vi "3D_Traverse_move.vi"(0 "Mode":T3=enum."Read traverse position", 1 "Route Checking?":bool=TRUE, 2 "Row Number":i32=-1, 5 "Position":dbl[](array[numeric])=[0.0, 0.0, 0.0] format="%#.2f", 7 "Work in Tunnel Coordinates":T1, 11 "Simulate/Run":T2=enum."Run VI", 12 "Traverse name":string, 13 "Backlash Compensation?":bool=TRUE, 14 "Currently on Point":i32=-1) -> (3 "Model Rotation (deg)":dbl format="%#.2f", 4 "Trav Position achieved":dbl[](array[numeric]) format="%#.2f", 15 "Error String":string)   [LabVIEW 2010]
uses:
  Trav_mode.ctl
  Controls/User_Specific_mode.ctl
  Controls/Tunnel_Coordinates.ctl
  Route mapping/Route_Display_Mode.ctl
  Controls/In_Range.ctl
  Globals/Trav_pos_global.vi
  Globals/Constants_global.vi
  Route mapping/Route_mapping_global.vi
panel:
  in  "Position Increment":dbl[](array[numeric])=[0.0, 0.0, 0.0] step=0.1 format="%#.2f"
  out "Traverses Available":string[](array[string])
  in  "Traverse":u16(ring) items=["A_Tunnel", "Aero_Laser", "Aero_ThroughWall", "Aero_Tunnel", "Angle_Calibrator", "B_Tunnel", "D_Tunnel", "Dummy_Traverse", "EnFlo_Stack", "EnFlo_Tunnel", "EnFlo_Turntable", "Laser_Meas_Traverse", "mohd_setup", "Paul_Desk_Test", "PIV_Traverse"]
  # "X                Y                   Z"
  # "X                Y                   Z"
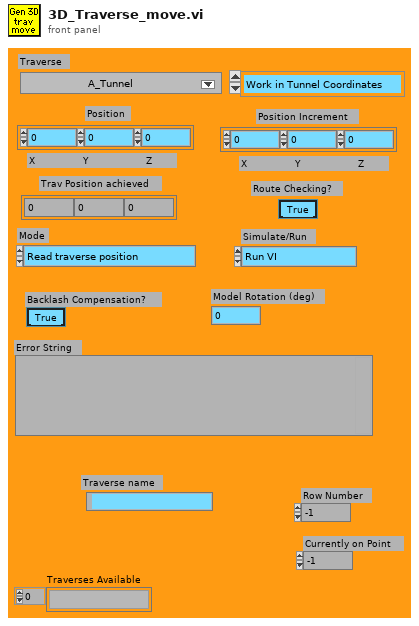
[diagram p1: front panel]
types:
  T1 = typedef "Tunnel_Coordinates.ctl" = enum16{"Work in Tunnel Coordinates", "Work in Model Coordinates"}
  T2 = typedef "User_Specific_mode.ctl" = enum16{"Check VI only", "Run VI"}
  T3 = typedef "Trav_mode.ctl" = enum16{"Move traverse", "Read traverse position", "Teach Position"}
  T4 = enum16{"To Traverse Coordinates", "To User Coordinates"}
  T5 = typedef "Route_Display_Mode.ctl" = enum16{"Display View Always", "Display View on Crash"}
  T6 = typedef "In_Range.ctl" = enum16{"%", "±", "% & ±"}
  T7 = typedef "Box_size.ctl" = cluster{"Max":dbl, "Min":dbl}[]
  T8 = typedef "Exclude_cluster.ctl" = cluster{"Sizes":T7, "Name":string, "Exclude Type":T9}
  T9 = typedef "Exclusion_type.ctl" = enum16{"Exclude completely", "Allow only vertical moves"}
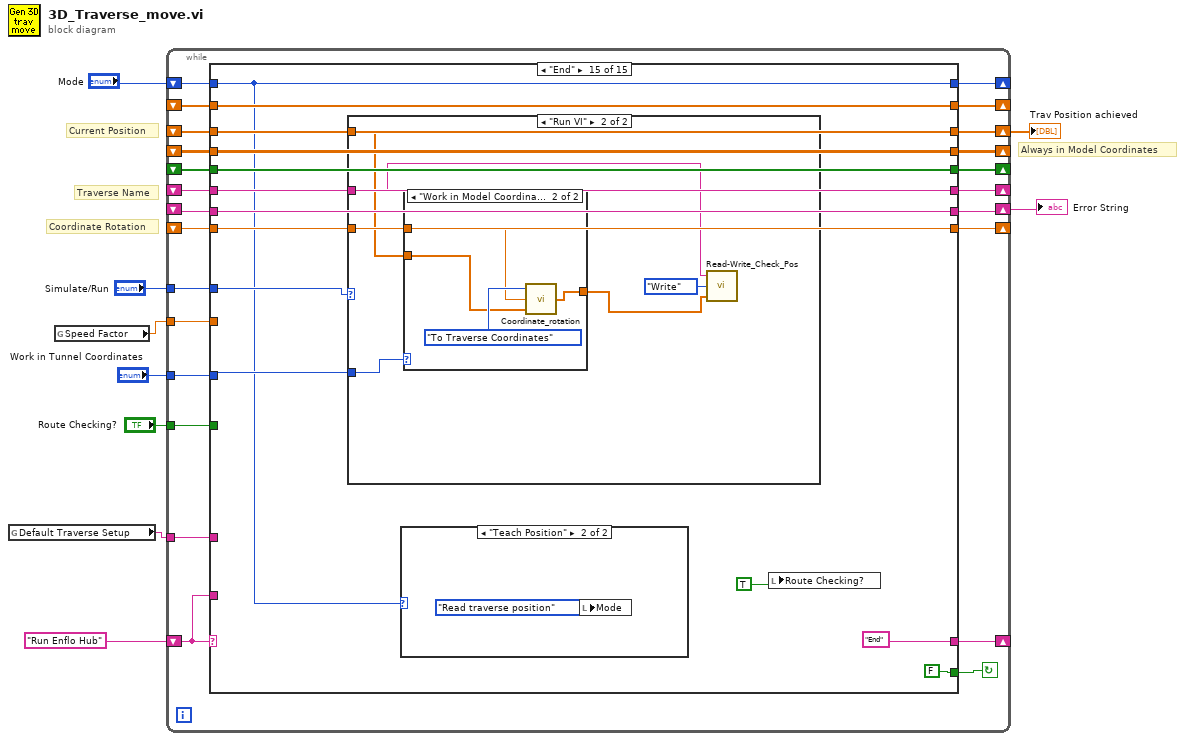
[diagram p0: block diagram]
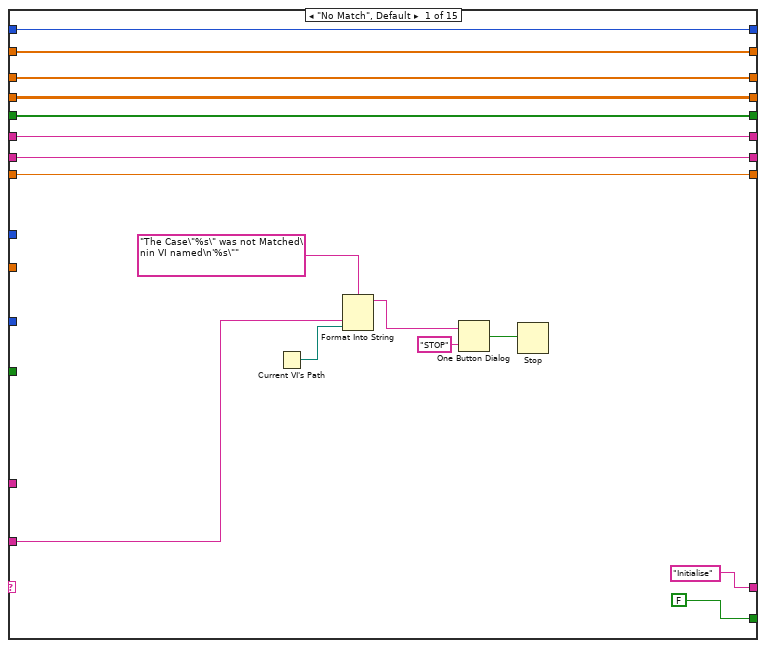
[diagram p2: hidden frame]
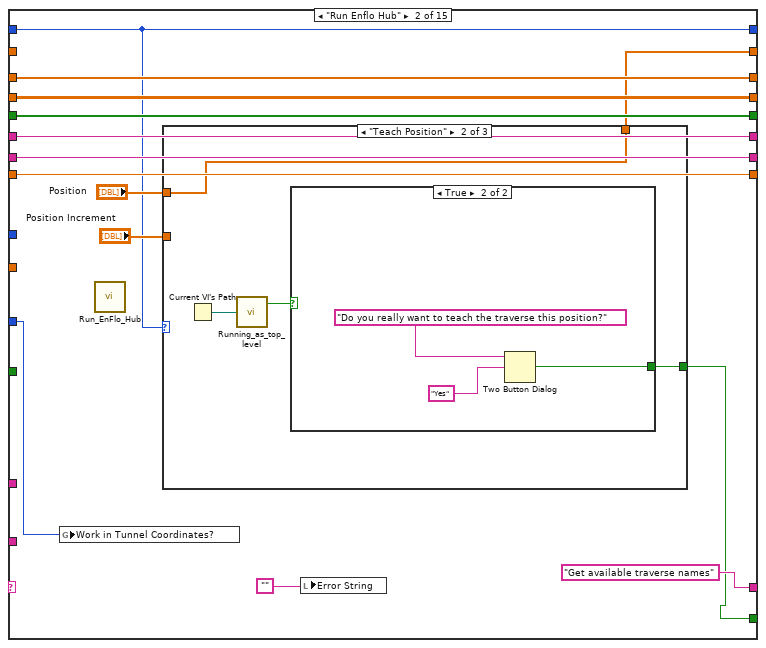
[diagram p3: hidden frame]
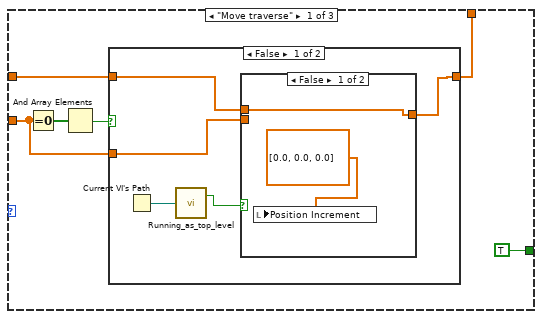
[diagram p4: hidden frame]
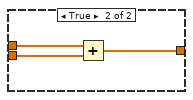
[diagram p5: hidden frame]
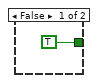
[diagram p7: hidden frame]
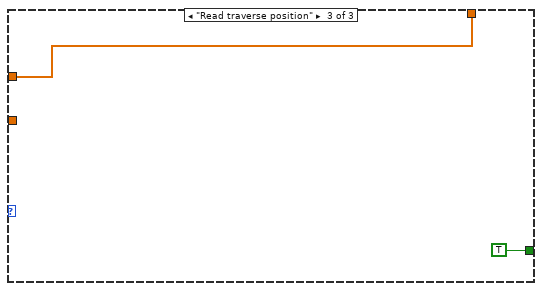
[diagram p8: hidden frame]
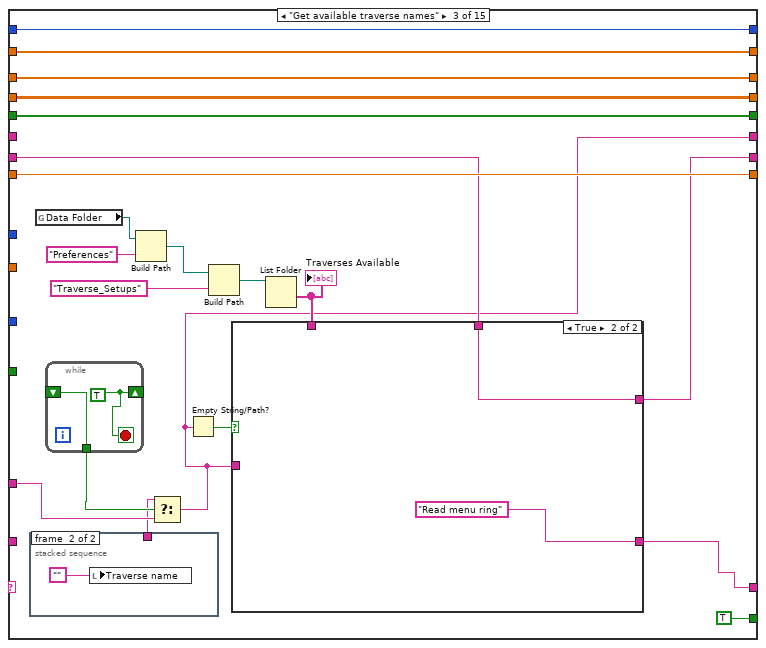
[diagram p9: hidden frame]
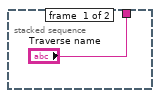
[diagram p10: hidden frame]
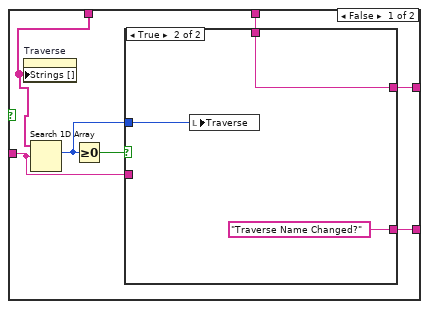
[diagram p11: hidden frame]
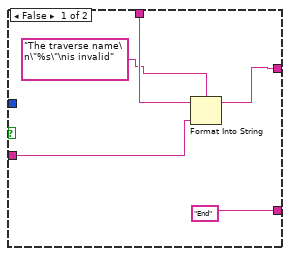
[diagram p12: hidden frame]
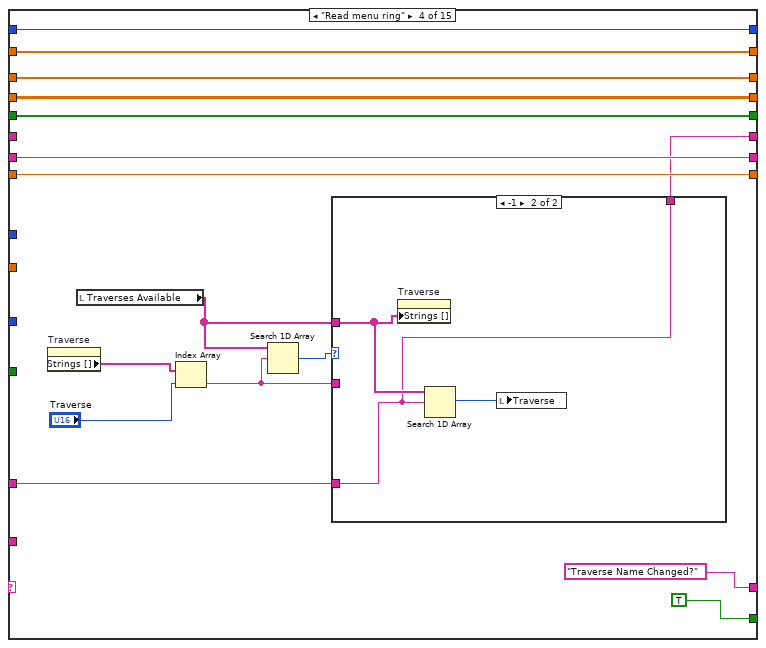
[diagram p13: hidden frame]
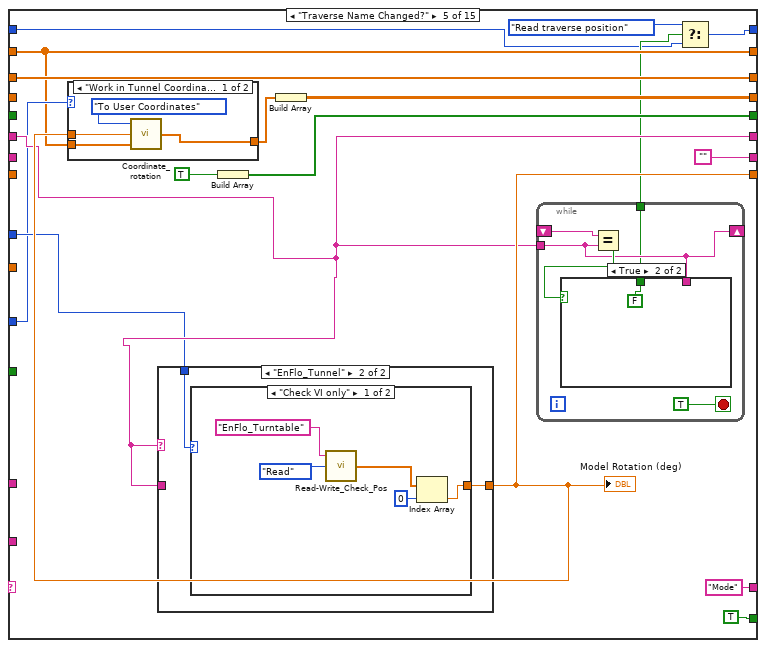
[diagram p15: hidden frame]
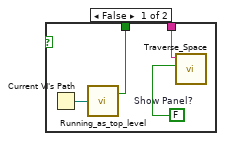
[diagram p17: hidden frame]
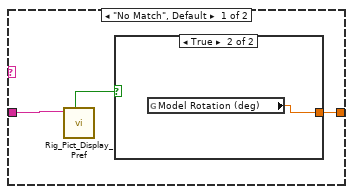
[diagram p18: hidden frame]
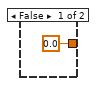
[diagram p19: hidden frame]
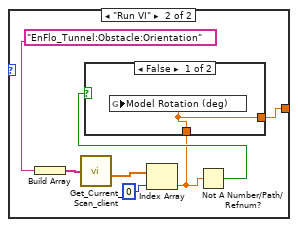
[diagram p20: hidden frame]
diagram:
  # "Always in Model Coordinates"
  # "Current Position"
  # "Coordinate Rotation"
  # "Traverse Name"
  n1 = global read "Trav_pos_global.vi" "Default Traverse Setup"() -> (w2:string)
  n2 = global read "Trav_pos_global.vi" "Speed Factor"() -> (w6:dbl)
  n3 = while {
    shift-left: "Run Enflo Hub" -> [w31]
    shift-right: [w32] -> _
    shift-right: [w29] -> _
    shift-left: _ -> [w27]
    tunnel: "Simulate/Run" -> [w30]
    shift-right: [w28] -> w7
    shift-left: _ -> [w26]
    shift-right: [w24] -> _
    shift-left: _ -> [w25]
    shift-right: [w19] -> _
    shift-left: _ -> [w18]
    shift-right: [w21] -> _
    shift-left: _ -> [w20]
    shift-right: [w22] -> w3
    shift-left: _ -> [w23]
    tunnel: w6 -> [w17]
    tunnel: "Work in Tunnel Coordinates" -> [w16]
    tunnel: "Route Checking?" -> [w15]
    tunnel: w2 -> [w14]
    shift-right: [w13] -> _
    shift-left: _ -> [w12]
    shift-right: [w10] -> _
    shift-left: "Mode" -> [w11]
    stop <- w33 continue-if-true
    n4 = case shown="\"End\"" w31 {
      tunnel: [FALSE w55 TRUE TRUE TRUE TRUE w266 TRUE ("T button?") TRUE w352 w372 TRUE TRUE TRUE FALSE] -> w33
      tunnel: ["Initialise" "Get available traverse names" w101 "Traverse Name Changed?" "Mode" w215 w255 "Perform Route Check" w316 "Display Traverse Views" w379 "Update Position Globals" "Tidy up" "End" "End"] -> w32
      tunnel: w31 -> [w44 _ _ _ _ _ _ _ _ _ _ _ _ _ _]
      tunnel: w30 -> [_ _ _ _ w159 w216 w260 _ w312 _ w377 _ _ _ w510]
      tunnel: [w41 w62 w94 w133 w160 w207 w268 w292 w311 w359 w384 w420 w445 w462 w506] -> w29
      tunnel: [w40 w61 w99 w146 "" w217 w267 "" w321 w349 w381 w409 w448 w464 w513] -> w28
      tunnel: w27 -> [w41 w62 _ _ w160 w207 w268 w292 w311 w359 w384 w420 w445 w462 w506]
      tunnel: w26 -> [w40 w61 w98 w146 _ w217 _ _ _ w350 w381 _ w448 w465 w513]
      tunnel: w25 -> [w39 w60 w111 w145 _ w218 w264 w295 w307 w358 w388 w416 w447 w468 w507]
      tunnel: [w39 w60 w111 w145 w162 w218 w264 w295 w307 w358 w388 w416 w447 w468 w507] -> w24
      tunnel: w23 -> [w38 w59 w110 w144 w165 w209 w261 _ w319 w357 w387 _ w444 w466 w508]
      tunnel: [w38 w59 w110 w144 w165 w209 w262 w294 w320 w357 w387 w414 w444 w466 w508] -> w22
      tunnel: [w37 w58 w109 w143 w166 w220 w270 w299 w318 w356 w385 w418 w449 w469 w514] -> w21
      tunnel: w20 -> [w37 w58 w109 w143 _ w220 w270 w299 _ w356 w385 w418 w449 w469 w514]
      tunnel: [w36 w57 w108 w142 w163 w219 w269 w298 w323 w355 w386 w412 w450 w470 w515] -> w19
      tunnel: w18 -> [w36 w57 w108 w142 _ w219 w269 w298 _ w355 w386 w412 w450 w470 w515]
      tunnel: w17 -> [_ _ _ _ _ _ _ _ _ _ _ w419 _ _ _]
      tunnel: w16 -> [_ w54 _ _ w158 w211 w265 w296 w329 _ _ w417 _ _ w509]
      tunnel: w15 -> [_ _ _ _ _ w212 _ _ _ _ _ w408 _ _ _]
      tunnel: w14 -> [_ _ w95 w137 _ _ _ _ _ _ _ _ _ _ _]
      tunnel: [w35 w53 w92 w135 w157 w208 w254 w293 w306 w348 w371 w407 w446 w461 w511] -> w13
      tunnel: w12 -> [w35 _ w92 w135 w157 w208 w254 w293 w306 w348 w371 w407 w446 w461 w511]
      tunnel: w11 -> [w34 w50 w91 w134 w153 w206 w253 w288 w305 w347 w370 w406 w443 w460 w505]
      tunnel: [w34 w50 w91 w134 w154 w206 w253 w288 w305 w347 w370 w406 w443 w460 w505] -> w10
      frame "No Match", Default {
        n5 = Current VI's Path() -> (path=w43:path)
        n6 = Format Into String(format string="The Case\"%s\" was not Matched\nin VI named\n'%s\"" ("Format String"), w44, w43) -> (resulting string=w47:string)  [unwired: 2 in, 1 out]
        n7 = One Button Dialog(message=w47, button name ("OK")="STOP") -> (true=w45:bool)
        n8 = Stop(stop? (T)=w45) -> ()
      }
      frame "Run Enflo Hub" {
        n9 = global write "Trav_pos_global.vi" "Work in Tunnel Coordinates?"(w54) -> ()
        n10 = call "Run_EnFlo_Hub.vi"() -> ()  [unwired: 8 out]
        n11 = case shown="\"Teach Position\"" w50 {
          tunnel: [TRUE ("T button?") w82 TRUE ("T button?")] -> w55
          tunnel: [w66 w81 w90] -> w53
          tunnel: "Position" -> [w65 w81 w90]
          tunnel: "Position Increment" -> [w64 _ _]
          frame "Move traverse" {
            n12 = Equal To 0?(x=w64) -> (x = 0?=w68:bool[])
            n13 = And Array Elements(Boolean array=w68) -> (logical AND=w67:bool)
            n14 = case shown="False" w67 {
              tunnel: [w70 w80] -> w66
              tunnel: w65 -> [w72 w80]
              tunnel: w64 -> [w71 _]
              frame False {
                n15 = Current VI's Path() -> (path=w74:path)
                n16 = call "Running_as_top_level.vi"("Vi path name"=w74) -> ("Top Level"=w73:bool)  [unwired: 1 out]
                n17 = case shown="False" w73 {
                  tunnel: w72 -> [w76 w79]
                  tunnel: w71 -> [_ w78]
                  tunnel: [w76 w77] -> w70
                  frame False {
                    n18 = local write "Position Increment"(dbl[] [0.0, 0.0, 0.0] ("Position Increment")) -> ()
                  }
                  frame True {
                    n19 = Add(x=w79, y=w78) -> (x+y=w77:dbl[])
                  }
                }
              }
              frame True {
              }
            }
          }
          frame "Teach Position" {
            n20 = Current VI's Path() -> (path=w84:path)
            n21 = call "Running_as_top_level.vi"("Vi path name"=w84) -> ("Top Level"=w83:bool)  [unwired: 1 out]
            n22 = case shown="True" w83 {
              tunnel: [TRUE ("T button?") w86] -> w82
              frame False {
              }
              frame True {
                n23 = Two Button Dialog(message="Do you really want to teach the traverse this position?", 2:"Yes" ("T button name (\"OK\")")) -> (T button?=w86:bool)  [unwired: 1 out]
              }
            }
          }
          frame "Read traverse position" {
          }
        }
        n24 = local write "Error String"("") -> ()
      }
      frame "Get available traverse names" {
        n25 = stacked-sequence {
          tunnel: ["Traverse name" _] -> w93
          frame #0 {
          }
          frame #1 {
            n26 = local write "Traverse name"("") -> ()
          }
        }
        n27 = global read "Constants_global.vi" "Data Folder"() -> (w104:path)
        n28 = while {
          shift-right: [w114] -> _
          shift-left: _ -> [w115]
          tunnel: [w115] -> w96
          stop <- w114 stop-if-true
          w114 = TRUE
        }
        n29 = Build Path(base path=w104, name or relative path="Preferences") -> (appended path=w106:path)
        n30 = Select(t=w93, s=w96, f=w95) -> (s? t:f=w94:string)
        n31 = Empty String/Path?(string/path=w94) -> (empty?=w102:bool)
        n32 = Build Path(base path=w106, name or relative path="Traverse_Setups") -> (appended path=w107:path)
        n33 = List Folder(path=w107) -> (folder names=w100:string[])  [unwired: 1 in, 5 out]
        "Traverses Available" <- w100
        n34 = case shown="True" w102 {
          tunnel: [w119 "Read menu ring"] -> w101
          tunnel: w100 -> [w116 _]
          tunnel: w94 -> [w122 _]
          tunnel: [w121 w131] -> w99
          tunnel: w98 -> [w120 w131]
          frame False {
            n35 = property on="Traverse" class="Ring (strict)"("Strings []"=w116) -> ()  [unwired: 2 in, 2 out]
            n36 = Search 1D Array(1D array=w116, element=w122) -> (index of element=w117:i32)  [unwired: 1 out]
            n37 = Greater Or Equal To 0?(x=w117) -> (x >= 0?=w118:bool)
            n38 = case shown="True" w118 {
              tunnel: w122 -> [w127 _]
              tunnel: [w124 w130] -> w121
              tunnel: w120 -> [w126 w130]
              tunnel: ["End" "Traverse Name Changed?"] -> w119
              tunnel: w117 -> [_ w128]
              frame False {
                n39 = Format Into String(format string="The traverse name\n\"%s\"\nis invalid", initial string=w126, w127) -> (resulting string=w124:string)  [unwired: 1 in, 1 out]
              }
              frame True {
                n40 = local write "Traverse"(w128) -> ()
              }
            }
          }
          frame True {
          }
        }
      }
      frame "Read menu ring" {
        n41 = property on="Traverse" class="Ring (strict)"() -> ("Strings []"=w141:string[])  [unwired: 2 in, 2 out]
        n42 = local read "Traverses Available"() -> (w138:string[])
        n43 = Index Array(array=w141, index="Traverse") -> (element=w136:string)
        n44 = Search 1D Array(1D array=w138, element=w136) -> (index of element=w139:i32)  [unwired: 1 out]
        n45 = case shown="-1" w139 {
          tunnel: w138 -> [_ w152]
          tunnel: w137 -> [_ w150]
          tunnel: [w149 w150] -> w133
          tunnel: w136 -> [w149 _]
          frame 0, Default {
          }
          frame -1 {
            n46 = property on="Traverse" class="Ring (strict)"("Strings []"=w152) -> ()  [unwired: 2 in, 2 out]
            n47 = Search 1D Array(1D array=w152, element=w150) -> (index of element=w151:i32)  [unwired: 1 out]
            n48 = local write "Traverse"(w151) -> ()
          }
        }
      }
      frame "Traverse Name Changed?" {
        n49 = case shown="\"EnFlo_Tunnel\"" w160 {
          tunnel: [w185 w191] -> w162
          tunnel: w159 -> [_ w190]
          tunnel: w160 -> [w187 _]
          frame "No Match", Default {
            n50 = call "Rig_Pict_Display_Pref.vi"("Traverse Name"=w187) -> ("Co-ordinate Transform"=w186:bool)  [unwired: 7 out]
            n51 = case shown="True" w186 {
              tunnel: [0.0 ("Model Rotation (deg)") w189] -> w185
              frame False {
              }
              frame True {
                n52 = global read "Trav_pos_global.vi" "Model Rotation (deg)"() -> (w189:dbl)
              }
            }
          }
          frame "EnFlo_Tunnel" {
            n53 = case shown="\"Check VI only\"" w190 {
              tunnel: [w192 w197] -> w191
              frame "Check VI only" {
                n54 = call "Read-Write_Check_Pos.vi"("Mode"=enum16{"Read", "Write"}."Read", "Traverse Name"="EnFlo_Turntable") -> ("Position Output"=w194:dbl[])  [unwired: 1 in]
                n55 = Index Array(array=w194, index=0) -> (element=w192:dbl)
              }
              frame "Run VI" {
                n56 = Build Array("EnFlo_Tunnel:Obstacle:Orientation") -> (w202:string[])
                n57 = call "Get_Current_Scan_client.vi"("ADAM Ch Names"=w202) -> ("Numerical Values"=w201:dbl[])  [unwired: 3 out]
                n58 = Index Array(array=w201, index=0) -> (element=w198:dbl)
                n59 = Not A Number/Path/Refnum?(number/path/refnum=w198) -> (NaN/Path/Refnum?=w199:bool)
                n60 = case shown="False" w199 {
                  tunnel: w198 -> [w204 _]
                  tunnel: [w204 w205] -> w197
                  frame False {
                    n61 = global write "Trav_pos_global.vi" "Model Rotation (deg)"(w204) -> ()
                  }
                  frame True {
                    n62 = global read "Trav_pos_global.vi" "Model Rotation (deg)"() -> (w205:dbl)
                  }
                }
              }
            }
          }
        }
        "Model Rotation (deg)" <- w162
        n63 = case shown="\"Work in Tunnel Coordinates\"" w158 {
          tunnel: w157 -> [w172 w174]
          tunnel: [w171 w174] -> w161
          tunnel: w162 -> [w170 _]
          frame "Work in Tunnel Coordinates" {
            n64 = call "Coordinate_rotation.vi"("Input Position"=w172, "Coordinate rotation (deg)"=w170, "Mode"=T4."To User Coordinates") -> ("Output Position"=w171:dbl[])
          }
          frame "Work in Model Coordinates" {
          }
        }
        n65 = Build Array(TRUE) -> (w163:bool[])
        n66 = Build Array(w161) -> (w166:dbl[][])
        n67 = while {
          shift-right: [w176] -> _
          shift-left: _ -> [w178]
          tunnel: w160 -> [w176]
          tunnel: [w175] -> w156
          stop <- TRUE stop-if-true
          n68 = Equal?(x=w178, y=w176) -> (x = y?=w177:bool)
          n69 = case shown="True" w177 {
            tunnel: w176 -> [w182 _]
            tunnel: [w180 FALSE ("Top Level")] -> w175
            frame False {
              w183 = FALSE  # Show Panel?
              n70 = Current VI's Path() -> (path=w181:path)
              n71 = call "Running_as_top_level.vi"("Vi path name"=w181) -> ("Top Level"=w180:bool)  [unwired: 1 out]
              n72 = call "Traverse_Space.vi"("Show Panel?"=w183, "Traverse Setup"=w182) -> ()  [unwired: 1 in, 8 out]
            }
            frame True {
            }
          }
        }
        n73 = Select(t=Trav_mode."Read traverse position" ("Mode"), s=w156, f=w153) -> (s? t:f=w154:T3)
      }
      frame "Mode" {
        n74 = while {
          shift-right: [w224] -> _
          shift-left: _ -> [w223]
          tunnel: w211 -> [w224]
          tunnel: [w222] -> w210
          stop <- TRUE stop-if-true
          n75 = Equal?(x=w223, y=w224) -> (x = y?=w222:bool)
        }
        n76 = case shown="\"Run VI\"" w216 {
          tunnel: w206 -> [_ w232]
          tunnel: [w226 w231] -> w215
          tunnel: "Execute case" -> [_ w230]
          tunnel: "Read Current Position" -> [w226 w229]
          tunnel: w212 -> [_ w228]
          tunnel: w210 -> [_ _]
          tunnel: w207 -> [_ w227]
          frame "Check VI only" {
          }
          frame "Run VI" {
            n77 = case shown="\"Move traverse\"" w232 {
              tunnel: [w235 w252] -> w231
              tunnel: w230 -> [w234 w252]
              tunnel: w229 -> [w233 _]
              tunnel: w228 -> [w236 _]
              tunnel: w227 -> [w237 _]
              frame "Move traverse" {
                n78 = case shown="True" w236 {
                  tunnel: w237 -> [_ w248]
                  tunnel: [w238 w242] -> w235
                  tunnel: w234 -> [w238 _]
                  tunnel: w233 -> [_ w240]
                  frame False {
                  }
                  frame True {
                    n79 = global read "Constants_global.vi" "Traverse folder"() -> (w249:path)
                    n80 = Build Path(base path=w249, name or relative path=w248) -> (appended path=w251:path)
                    n81 = Build Path(base path=w251, name or relative path="Traverse_Pos.xls" ("Substring")) -> (appended path=w247:path)
                    n82 = File/Directory Info(path=w247) -> (last mod=w245:timestamp)  [unwired: 1 in, 6 out]
                    n83 = Get Date/Time In Seconds() -> (seconds since 1Jan1904=w246:timestamp)
                    n84 = Subtract(x=w246, y=w245) -> (x-y=w244:dbl)
                    n85 = Greater?(x=w244, y=40.0) -> (0:w241:bool)
                    n86 = Select(t=w240, s=w241, f="Quick Read from file") -> (s? t:f=w242:string)
                  }
                }
              }
              frame "Read traverse position", Default {
              }
            }
          }
        }
      }
      frame "Read Current Position" {
        n87 = case shown="\"Run VI\"" w260 {
          tunnel: w268 -> [w271 w280]
          tunnel: ["" w282] -> w267
          tunnel: w264 -> [_ w275]
          tunnel: [w272 w281] -> w263
          tunnel: w261 -> [_ w277]
          frame "Check VI only" {
            n88 = call "Read-Write_Check_Pos.vi"("Mode"=enum16{"Read", "Write"}."Read", "Traverse Name"=w271) -> ("Position Output"=w272:dbl[])  [unwired: 1 in]
          }
          frame "Run VI" {
            w279 = FALSE  # Route Checking?
            w278 = FALSE  # Backlash Compensation?
            n89 = call "TraverseControl.vi"("Mode"=Trav_mode."Read traverse position", "Route Checking?"=w279, "Traverse Name"=w280, "Coordinate rotation (deg)"=w275, "Position input XYZ"=w277, "Backlash Compensation?"=w278) -> ("Position Output XYZ"=w281:dbl[], "Error String"=w282:string)  [unwired: 1 in, 7 out]
          }
        }
        n90 = Equal?(x=Trav_mode."Read traverse position" ("Mode"), y=w253) -> (x = y?=w258:bool)
        n91 = case shown="\"Work in Model Coordinates\"" w265 {
          tunnel: w263 -> [w283 w286]
          tunnel: [w283 w285] -> w262
          tunnel: w264 -> [_ w284]
          frame "Work in Tunnel Coordinates" {
          }
          frame "Work in Model Coordinates" {
            n92 = call "Coordinate_rotation.vi"("Input Position"=w286, "Coordinate rotation (deg)"=w284, "Mode"=T4."To User Coordinates") -> ("Output Position"=w285:dbl[])
          }
        }
        n93 = Empty String/Path?(string/path=w267) -> (empty?=w266:bool)
        n94 = Select(t="Update Position Globals", s=w258, f="Perform Route Check") -> (s? t:f=w255:string)
      }
      frame "Quick Read from file" {
        n95 = call "Read_Traverse_Pos_File.vi"("Traverse Name"=w292) -> ("Tunnel Coordinates"=w291:dbl[])
        n96 = case shown="\"Work in Model Coordinates\"" w296 {
          tunnel: w291 -> [w300 w303]
          tunnel: [w300 w302] -> w294
          tunnel: w295 -> [_ w301]
          frame "Work in Tunnel Coordinates" {
          }
          frame "Work in Model Coordinates" {
            n97 = call "Coordinate_rotation.vi"("Input Position"=w303, "Coordinate rotation (deg)"=w301, "Mode"=T4."To User Coordinates") -> ("Output Position"=w302:dbl[])
          }
        }
      }
      frame "Perform Route Check" {
        n98 = case shown="\"Work in Tunnel Coordinates\"" w329 {
          tunnel: w307 -> [w343 _]
          tunnel: w306 -> [w339 w345]
          tunnel: w319 -> [w342 w346]
          tunnel: [w341 w345] -> w310
          tunnel: [w340 w346] -> w322
          frame "Work in Tunnel Coordinates" {
            w344 = T4."To User Coordinates" ("Mode")
            n99 = call "Coordinate_rotation.vi"("Input Position"=w342, "Coordinate rotation (deg)"=w343, "Mode"=w344) -> ("Output Position"=w340:dbl[])
            n100 = call "Coordinate_rotation.vi"("Input Position"=w339, "Coordinate rotation (deg)"=w343, "Mode"=w344) -> ("Output Position"=w341:dbl[])
          }
          frame "Work in Model Coordinates" {
          }
        }
        n101 = global read "Route_mapping_global.vi" "Entire Space"() -> (w328:T7)
        n102 = global read "Route_mapping_global.vi" "Exclude Array"() -> (w326:T8[])
        n103 = global read "Route_mapping_global.vi" "Probe Volume"() -> (w327:T7)
        n104 = call "Check_with_Jump.vi"("Rotation (deg)"=w307, "Simulate/Run"=w312, "Exclude Array"=w326, "Traverse Name"=w311, "Probe Volume"=w327, "Entire Space"=w328, "New Position"=w310, "Current position"=w322) -> ("Steps"=w318:dbl[][], "Error Comments"=w321:string)  [unwired: 2 out]
        n105 = Array Size(array=w318) -> (size(s)=w325:i32[])
        n106 = Empty String/Path?(string/path=w321) -> (empty?=w313:bool)
        n107 = case shown="True" w313 {
          tunnel: [w337 w338] -> w320
          tunnel: w319 -> [w337 _]
          tunnel: w306 -> [_ w338]
          frame False {
          }
          frame True {
          }
        }
        n108 = Index Array(array=w325, index=0) -> (element=w308:i32)
        n109 = case shown="3, Default" w308 {
          tunnel: [w331 w333 w336] -> w323
          tunnel: "Backlash Compensation?" -> [w330 w332 w334]
          frame 1 {
            n110 = Build Array(w330) -> (w331:bool[])
          }
          frame 2 {
            n111 = Build Array(w332, w332) -> (w333:bool[])
          }
          frame 3, Default {
            n112 = Build Array(FALSE, w334, w334) -> (w336:bool[])
          }
        }
        n113 = Select(t="Display Traverse Views", s=w313, f="Route Error") -> (s? t:f=w316:string)
      }
      frame "Route Error" {
        n114 = global read "Trav_pos_global.vi" "Jump Bad Positions?"() -> (w354:bool)
        n115 = case shown="True" w354 {
          tunnel: w348 -> [_ w362]
          tunnel: [TRUE w361] -> w352
          frame False {
          }
          frame True {
            n116 = Current VI's Path() -> (path=w364:path)
            n117 = call "Running_as_top_level.vi"("Vi path name"=w364) -> ("Top Level"=w363:bool)  [unwired: 1 out]
            n118 = case shown="False" w363 {
              tunnel: w362 -> [w366 _]
              tunnel: [FALSE TRUE] -> w361
              frame False {
                n119 = global read "Trav_pos_global.vi" "Jumped Positions"() -> (w365:dbl[][])
                n120 = Build Array (concatenate)(w366, w365) -> (w368:dbl[][])
                n121 = global write "Trav_pos_global.vi" "Jumped Positions"(w368) -> ()
              }
              frame True {
              }
            }
          }
        }
        n122 = Concatenate Strings("Route Checking Error\n" ("string"), w350) -> (w349:string)
      }
      frame "Display Traverse Views" {
        n123 = global read "Route_mapping_global.vi" "Display Mode"() -> (w383:T5)
        n124 = Equal?(x=w377, y=User_Specific_mode."Check VI only" ("Simulate/Run")) -> (x = y?=w376:bool)
        n125 = Empty String/Path?(string/path=w381) -> (empty?=w372:bool)
        n126 = Equal?(x=w383, y=Route_Display_Mode."Display View Always" ("Display Mode")) -> (x = y?=w380:bool)
        n127 = Not(x=w372) -> (.not. x?=w373:bool)
        n128 = Or(x=w380, y=w373) -> (x .or. y?=w375:bool)
        n129 = And(x=w376, y=w375) -> (x .and. y?=w374:bool)
        n130 = case shown="True" w374 {
          tunnel: w385 -> [_ w397]
          tunnel: w384 -> [_ w396]
          tunnel: w381 -> [_ w393]
          tunnel: w372 -> [_ w391]
          frame False {
          }
          frame True {
            n131 = Not(x=w391) -> (.not. x?=w392:bool)
            n132 = for {
              tunnel: w397 -> [w404] mode=indexing
              tunnel: w396 -> [w403]
              tunnel: "Currently on Point" -> [w402]
              tunnel: "Row Number" -> [w401]
              tunnel: w393 -> [w400]
              tunnel: w392 -> [w398]
              n133 = Build Array(w404) -> (w405:dbl[][])
              n134 = call "Display_Trav_Views.vi"("Current Probe Position"=w405, "Traverse Name"=w403, "Currently on point"=w402, "Open Front Panel"=TRUE, "Error Comments"=w400, "Crash?"=w398, "Row Number"=w401) -> ()  [unwired: 4 out]
            }
          }
        }
        n135 = case shown="\"Check VI only\"" w377 {
          tunnel: ["Update Position Globals" "Execute case"] -> w379
          frame "Check VI only" {
          }
          frame "Run VI" {
          }
        }
      }
      frame "Execute case" {
        n136 = Array Size(array=w412) -> (size(s)=w411:i32)
        n137 = Decrement(x=w411) -> (x-1=w410:i32)
        n138 = while {
          tunnel: w420 -> [w425]
          tunnel: w418 -> [w437] mode=indexing
          tunnel: w419 -> [w424]
          tunnel: w406 -> [w427]
          tunnel: w416 -> [w428]
          tunnel: [w430] -> w415
          tunnel: w412 -> [w423] mode=indexing
          tunnel: w410 -> [w434]
          tunnel: [w422] -> w409
          tunnel: w408 -> [w426]
          i -> [w435]
          stop <- w431 continue-if-true
          n139 = call "Coordinate_rotation.vi"("Input Position"=w437, "Coordinate rotation (deg)"=w428, "Mode"=T4."To Traverse Coordinates") -> ("Output Position"=w429:dbl[])
          n140 = Less?(x=w435, y=w434) -> (x < y?=w433:bool)
          n141 = call "TraverseControl.vi"("Mode"=w427, "Route Checking?"=w426, "Traverse Name"=w425, "Coordinate rotation (deg)"=w428, "Position input XYZ"=w429, "Speed Factor"=w424, "Backlash Compensation?"=w423) -> ("Position Output XYZ"=w430:dbl[], "Error String"=w422:string)  [unwired: 7 out]
          n142 = Empty String/Path?(string/path=w422) -> (empty?=w432:bool)
          n143 = And(x=w432, y=w433) -> (x .and. y?=w431:bool)
        }
        n144 = case shown="\"Work in Model Coordinates\"" w417 {
          tunnel: w415 -> [w438 w441]
          tunnel: [w438 w440] -> w414
          tunnel: w416 -> [_ w439]
          frame "Work in Tunnel Coordinates" {
          }
          frame "Work in Model Coordinates" {
            n145 = call "Coordinate_rotation.vi"("Input Position"=w441, "Coordinate rotation (deg)"=w439, "Mode"=T4."To User Coordinates") -> ("Output Position"=w440:dbl[])
          }
        }
      }
      frame "Update Position Globals" {
        n146 = case shown="\"Move traverse\", Default" w443 {
          tunnel: w445 -> [w455 _]
          tunnel: w444 -> [w453 _]
          frame "Move traverse", Default {
            n147 = Equal?(x="EnFlo_Turntable" ("y"), y=w455) -> (x = y?=w454:bool)
            n148 = case shown="True" w454 {
              tunnel: w453 -> [_ w457]
              frame False {
              }
              frame True {
                w459 = 0  # index
                n149 = Index Array(array=w457, index=w459) -> (element=w458:dbl)
                n150 = global write "Trav_pos_global.vi" "Model Rotation (deg)"(w458) -> ()
              }
            }
          }
          frame "Read traverse position" {
          }
        }
        n151 = local write "Position"(w444) -> ()
        n152 = global write "Trav_pos_global.vi" "Traverse position"(w444) -> ()
      }
      frame "Tidy up" {
        n153 = case shown="\"Read traverse position\", Default" w460 {
          tunnel: w466 -> [w475 w504]
          tunnel: w465 -> [w476 w503]
          tunnel: w461 -> [w474 _]
          tunnel: [w473 w503] -> w464
          frame "Move traverse" {
            n154 = Empty String/Path?(string/path=w476) -> (empty?=w477:bool)
            n155 = case shown="True" w477 {
              tunnel: w475 -> [_ w482]
              tunnel: w474 -> [_ w481]
              tunnel: w476 -> [w478 w480]
              tunnel: [w478 w479] -> w473
              frame False {
              }
              frame True {
                n156 = for {
                  tunnel: w482 -> [w485] mode=indexing
                  tunnel: w481 -> [w486] mode=indexing
                  shift-right: [w483] -> w479
                  shift-left: w480 -> [w484]
                  i -> [w489]
                  w491 = 10.0  # ±
                  n157 = case shown="0, Default" w489 {
                    tunnel: ["X" "Y" "Z"] -> w487
                    frame 0, Default {
                    }
                    frame 1 {
                    }
                    frame 2 {
                    }
                  }
                  n158 = call "In_Range_check.vi"("±"=w491, "Mode"=In_Range."±", "Value"=w486, "Setpoint"=w485) -> ("In Range"=w488:bool)  [unwired: 1 in, 2 out]
                  n159 = case shown="False" w488 {
                    tunnel: w487 -> [w498 _]
                    tunnel: w486 -> [w497 _]
                    tunnel: w485 -> [w496 _]
                    tunnel: w484 -> [w493 w499]
                    tunnel: [w494 w499] -> w483
                    frame False {
                      n160 = Format Into String(format string="For %s Axis Dem Pos = %.1f Achieved Pos = %.1f mm" ("Format String"), w498, w497, w496) -> (resulting string=w492:string)  [unwired: 2 in, 1 out]
                      n161 = Concatenate Strings(w493, w492) -> (w494:string)
                    }
                    frame True {
                    }
                  }
                }
              }
            }
          }
          frame "Read traverse position", Default {
            n162 = local write "Position"(w504) -> ()
          }
        }
        n163 = local write "Currently on Point"(-1 ("Row Number")) -> ()
        n164 = local write "Simulate/Run"(User_Specific_mode."Run VI" ("Simulate/Run")) -> ()
      }
      frame "End" {
        n165 = case shown="\"Run VI\"" w510 {
          tunnel: w509 -> [_ w523]
          tunnel: w508 -> [_ w520]
          tunnel: w507 -> [_ w519]
          tunnel: w506 -> [_ w518]
          frame "Check VI only", Default {
          }
          frame "Run VI" {
            n166 = case shown="\"Work in Model Coordinates\"" w523 {
              tunnel: w520 -> [w524 w527]
              tunnel: [w524 w526] -> w521
              tunnel: w519 -> [_ w525]
              frame "Work in Tunnel Coordinates" {
              }
              frame "Work in Model Coordinates" {
                n167 = call "Coordinate_rotation.vi"("Input Position"=w527, "Coordinate rotation (deg)"=w525, "Mode"=T4."To Traverse Coordinates") -> ("Output Position"=w526:dbl[])
              }
            }
            n168 = call "Read-Write_Check_Pos.vi"("Position input"=w521, "Mode"=enum16{"Read", "Write"}."Write", "Traverse Name"=w518) -> ()  [unwired: 1 out]
          }
        }
        n169 = case shown="\"Teach Position\"" w505 {
          frame "Move traverse", Default {
          }
          frame "Teach Position" {
            n170 = local write "Mode"(Trav_mode."Read traverse position" ("Mode")) -> ()
          }
        }
        n171 = local write "Route Checking?"(TRUE ("Route Checking?")) -> ()
      }
    }
  }
  "Trav Position achieved" <- w3
  "Error String" <- w7
